vi "RegisterLicense.vi"(7 "key":string, 8 "licensee":string, 10 "error in":errorcluster) -> (0 "State message":string, 1 "State":i32(ring) items=["Invalid", "Trial", "ExtraTrial", "Expired", "MaintenanceNeeded", "Licensed"], 3 "error out":errorcluster)   [LabVIEW 2022 SP3, in "UnderAutomation.UniversalRobots.lvlib"]
uses:
  UnderAutomation.UniversalRobots.lvlib
  C:/Users/fg/Documents/UniversalRobots.vi/LabVIEW_2024/UnderAutomation.UniversalRobots/lib/UnderAutomation.UniversalRobots.dll
  LabVIEW_2024/UnderAutomation.UniversalRobots/lib/UnderAutomation.UniversalRobots.dll
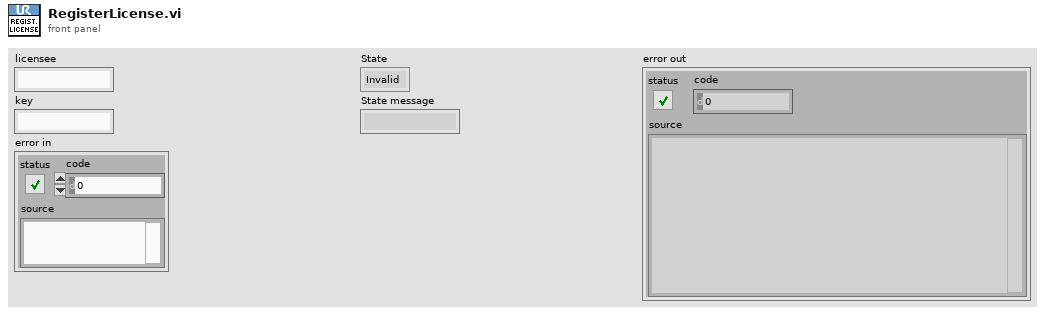
[diagram p1: front panel]
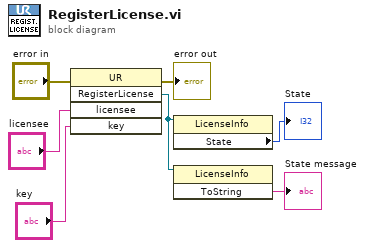
[diagram p0: block diagram]
diagram:
  n1 = invoke class="UR" method="RegisterLicense"(error in="error in", "licensee"="licensee", "key"="key") -> (error out=→"error out":errorcluster, "RegisterLicense"=w2:refnum<k24>)  [unwired: 2 in, 3 out]
  n2 = property class="LicenseInfo"(reference=w2) -> ("State"=→"State":i32)  [unwired: 1 in, 2 out]
  n3 = invoke class="LicenseInfo" method="ToString"(reference=w2) -> ("ToString"=→"State message":string)  [unwired: 2 in, 2 out]
